vi "LVClass_ComputePhaseSet GetTypePhase.vi"(0 "ComputePhaseSet in":refnum<class "ComputePhaseSet.lvclass">, 11 "error in (no error)":errorcluster) -> (4 "ComputePhaseSet out":refnum<class "ComputePhaseSet.lvclass">, 6 "Reconstruction Mode":T1=enum."Modal_Legendre", 15 "error out":errorcluster)   [LabVIEW 2020, in "ComputePhaseSet.lvclass"]
doc: "Get preferences for zonal phase reconstruction.\n\n--------------------------------------------------------------------------------\n\n<B>ComputePhaseSetIn </B> : ComputePhaseSet object.\n<B>ComputePhaseSetOut </B> : ComputePhaseSet object.\n<B>nb_weak_iterations </B> : Maximum number of weak iterations. A weak iteration is defined as an iteration\n for which the variation of the residue from previous iteration is below the\n residual_limit multiplied by the number of microlenses of the Haso.\n<B>nb_max_iterations </B> : Maximum number of iterations.\n<B>residual_limit </B> : Residual variation limit.\n<B>ErrorIn </B> : Error\n<B>ErrorOut </B> : Error\n\n--------------------------------------------------------------------------------"
uses:
  ComputePhaseSet.lvclass
  WavefrontReconstructionMode.ctl
  ComputePhaseSet.lvclass/ComputePhaseSet.ctl
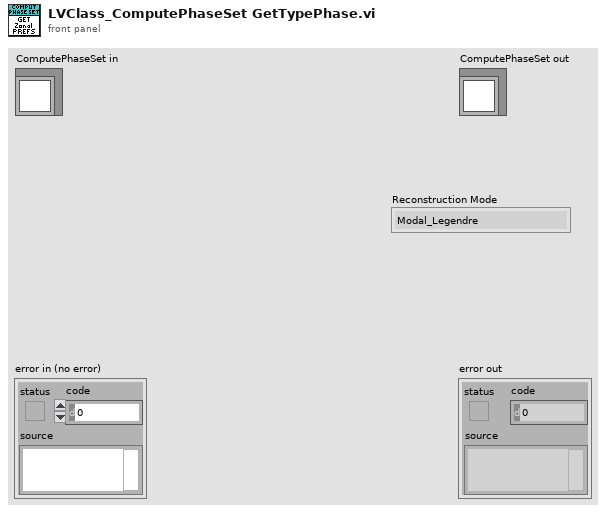
[diagram p1: front panel]
types:
  T1 = typedef "WavefrontReconstructionMode.ctl" = enum16{"None", "Modal_Legendre", "Modal_Zernike", "Zonal", "Modal_Zonal_Zernike", "Modal_Zonal_Legendre"}
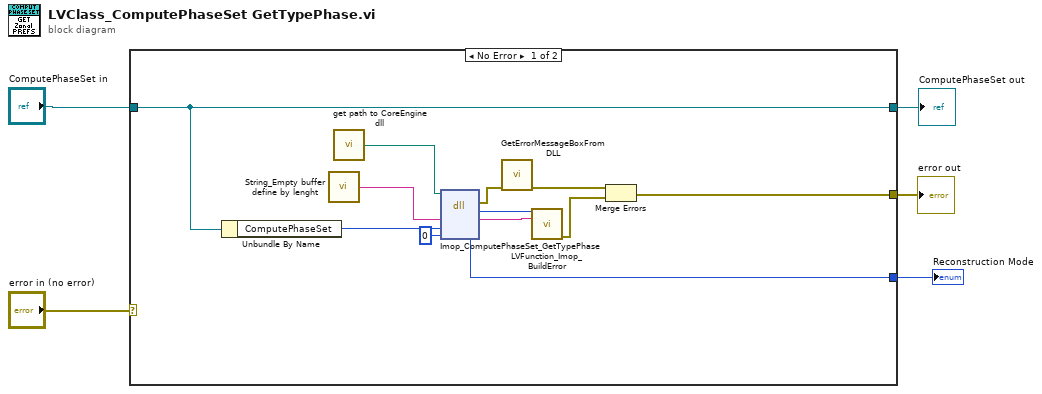
[diagram p0: block diagram]
diagram:
  n1 = case shown="No Error" "error in (no error)" {
    selector: "error in (no error)" -> [_ w19]
    tunnel: [w7 w19] -> w2
    tunnel: [w11 w18] -> w4
    tunnel: "ComputePhaseSet in" -> [w11 w18]
    tunnel: [w6 _] -> w1
    frame No Error {
      n2 = Unbundle By Name(w11) -> ("ComputePhaseSet"=w10:i32)
      n3 = call "String_Empty buffer define by lenght.vi"() -> ("Empty buffer"=w15:string)  [unwired: 1 in]
      n4 = call "get path to CoreEngine dll.vi"() -> ("path to c_interface_vc100.dll"=w14:path)  [unwired: 12 in, 3 out]
      n5 = dll-call lib="D:/2_trunk/Soft_haso/ImOpCoreEngine4_LV2011/DLLs/ImopEngine4_vc100.dll" fn="Imop_ComputePhaseSet_GetTypePhase"(path in=w14, "message"=w15, "ComputePhaseSet"=w10, "TypePhase"=u32 0 ("nb_weak_iterations")) -> (error out=w13:errorcluster, "return type"=w17:i32, "message"=w16:string, "TypePhase"=w6:u8)  [unwired: 3 in, 1 out]
      n6 = call "GetErrorMessageBoxFromDLL.vi"("error IN"=w13) -> ("error OUT"=w9:errorcluster)  [unwired: 10 in]
      n7 = call "LVFunction_Imop_BuildError.vi"("code"=w17, "String to Prepend to source (\"\")"=w16) -> ("error out"=w8:errorcluster)  [unwired: 13 in]
      n8 = Merge Errors(w9, w8) -> (w7:errorcluster)
    }
    frame Error {
    }
  }
  "error out" <- w2
  "ComputePhaseSet out" <- w4
  "Reconstruction Mode" <- w1
